vi "example_data_queue_1.vi"() -> ()   [LabVIEW 2015]
panel:
  in  "stop":bool
  out "Waveform Graph":dbl[][](graph)
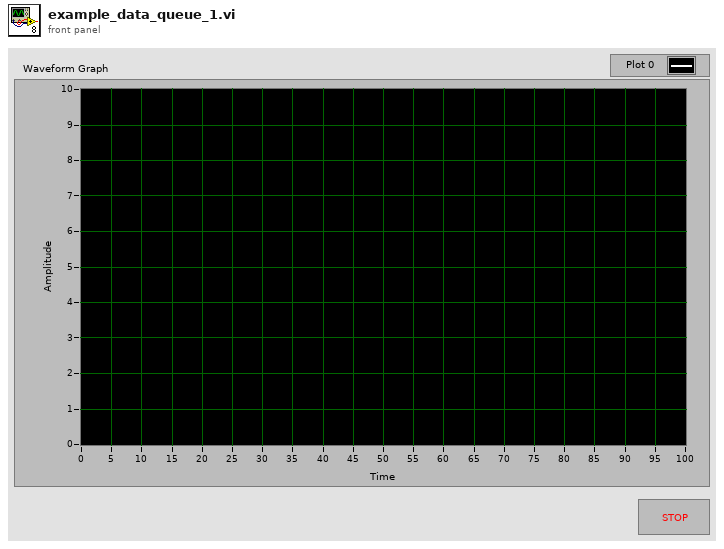
[diagram p1: front panel]
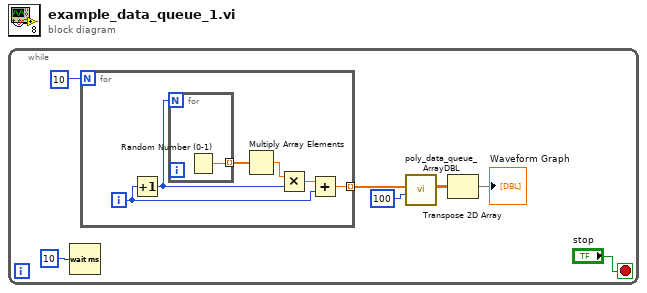
[diagram p0: block diagram]
diagram:
  n1 = while {
    stop <- "stop" stop-if-true
    n2 = Wait (ms)(milliseconds to wait=u32 10) -> ()  [unwired: 1 out]
    n3 = for {
      N: 10 -> [_]
      tunnel: [w12] -> w6 mode=indexing
      i -> [w11]
      n4 = Increment(x=w11) -> (x+1=w8:i32)
      n5 = for {
        N: w8 -> [_]
        tunnel: [w14] -> w13 mode=indexing
        n6 = Random Number (0-1)() -> (number: 0 to 1=w14:dbl)
      }
      n7 = Multiply Array Elements(1:w13) -> (0:w10:dbl)
      n8 = Multiply(x=w10, y=w8) -> (x*y=w9:dbl)
      n9 = Add(x=w9, y=w11) -> (x+y=w12:dbl)
    }
    n10 = call "poly_data_queue_ArrayDBL.vi"("queue length (100)"=100, "input data element"=w6) -> ("queue"=w5:dbl[][])  [unwired: 6 in, 3 out]
    n11 = Transpose 2D Array(2D array=w5) -> (transposed array=→"Waveform Graph":dbl[][])
  }
